vi "Write Cell String.vi"(8 "error in":errorcluster, 9 "Write to Cell":string, 10 "Cell Name":string, 11 "NI_report in":refnum<class "NI_report.lvclass">) -> (0 "error out":errorcluster, 3 "NI_report out":refnum<class "NI_report.lvclass">)   [LabVIEW 2015]
uses:
  <vilib>/Utility/NIReport.llb/NI_report.lvclass
  <vilib>/Utility/NIReport.llb/Append Report Text (str wrap).vi
  <vilib>/addons/_office/NI_ReportGenerationToolkit.lvlib
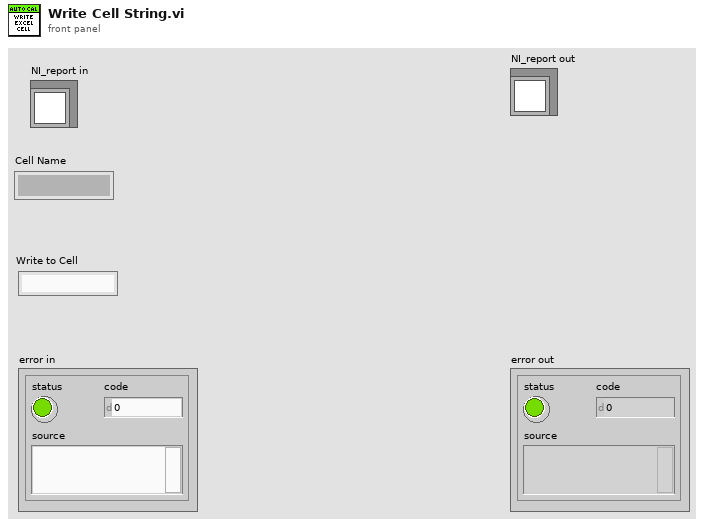
[diagram p1: front panel]
types:
  T1 = cluster{"position (excel)":cluster{"row":i32, "column":i32}, "name (excel)":string, "bookmark (word)":string}
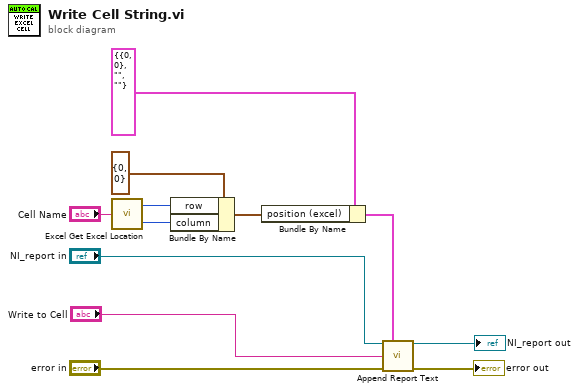
[diagram p0: block diagram]
diagram:
  n1 = call <vilib>:"Excel Get Excel Location.vi"("cell's name"="Cell Name") -> ("row"=w7:i32, "column"=w8:i32)
  n2 = Bundle By Name(cluster=cluster{"row":i32, "column":i32} {"row"=0, "column"=0} ("position (excel)"), "row"=w7, "column"=w8) -> (w9:cluster{"row":i32, "column":i32})
  n3 = Bundle By Name(cluster=T1 {"position (excel)"={"row"=0, "column"=0}, "name (excel)"="", "bookmark (word)"=""} ("MS Office parameters"), "position (excel)"=w9) -> (w10:T1)
  n4 = call-poly <vilib>:"Append Report Text.vi"("report in"="NI_report in", "MS Office parameters"=w10, "text"="Write to Cell", "error in (no error)"="error in") -> ("report out"=→"NI_report out":refnum<class "NI_report.lvclass">, "error out"=→"error out":errorcluster)  [unwired: 8 in, 2 out]
